vi "Fpga-FPGANic-Top.vi"() -> ()   [LabVIEW 2017]
uses:
  <instrlib>/_niInstr/Network/Ethernet/MAC/CLIP/v1/Resources.ctl
  <vilib>/Platform/TimedLoop/XDataNode/timing_clust.ctl
  <vilib>/Platform/TimedLoop/XDataNode/nitl_modes.ctl
  <vilib>/Platform/TimedLoop/XDataNode/wakeup.ctl
  FPGANic.Read.States.ctl
  <instrlib>/_niInstr/Network/Ethernet/MAC/Raw Stream/v1/niInstr Ethernet MAC Raw Stream v1.lvclass
  <instrlib>/_niInstr/Network/Ethernet/Utility/v1/FPGA/Network Data Stream.ctl
  FPGANic.Write.States.ctl
  <vilib>/rvi/Emulation/niFpgaSctlEmulationGetInTimedLoop.vi
  <vilib>/rvi/Emulation/niFpgaEmulationReportErrorSimple.vi
  <vilib>/rvi/Emulation/niFpgaGetClockAttributes.vi
  <vilib>/rvi/Emulation/niFpgaCriticalErrorInLSC.vi
  <vilib>/rvi/eio/common/nirviEmuTemplateMethod_errors.vi
  <vilib>/rvi/interface/RandomDataEmulation/niFpgaRandomDataHandleErrors.vi
  <vilib>/rvi/DataTransferAndStorage/Container/Common/niFpgaContainerGetUniqueNameForEmu.vi
  <vilib>/rvi/DataTransferAndStorage/Container/Common/niFpgaContainerSetEmuInfo.vi
  <vilib>/rvi/eio/common/nirviEmuReportErrorAndStop.vi
  <vilib>/rvi/DataTransferAndStorage/Container/Common/niFpgaContainerExecOnDevCompGetState.vi
  <vilib>/rvi/Emulation/niFpgaEmulationIsFPGAContextNoSignature.vi
  <vilib>/rvi/errors/niFpgaSetErrorForExecOnDevCompSimple.vi
  <vilib>/rvi/FIFO/Fifo_Resource/nirvififoEmulationSetSize.vi
  <vilib>/rvi/FIFO/Fifo_Resource/nirviFifoEmulationQueueMgr.vi
  <instcachedir>/0/nirviFifoEmulationQueueMgr_E5CAEC123FF24DC58D834DCA3CDAA9B5.lvgen/nirviFifoEmulationQueueMgr_E5CAEC123FF24DC58D834DCA3CDAA9B5_008.vi
  <vilib>/rvi/FIFO/Fifo_Resource/nirvififoEmulationDetermineInputValidOut.vi
  <vilib>/rvi/FIFO/Fifo_Resource/nirvififoEmulationCreateLock.vi
  <vilib>/rvi/Emulation/niFpgaProcessEmulError.vi
  <vilib>/rvi/FIFO/Fifo_Resource/nirvififoEmulationObtainLock.vi
  <vilib>/rvi/FIFO/Fifo_Resource/nirvififoEmulationReleaseLock.vi
  <vilib>/rvi/occurrence/nirviWaitOnOccurrenceBase.vi
  <vilib>/rvi/errors/nirviReportUnexpectedCaseInternalError.vi
  <vilib>/rvi/errors/nirviReportUnexpectedCaseInternalError (U32).vi
  <vilib>/Utility/error.llb/Clear Errors.vi
  <instrlib>/_niInstr/Network/Ethernet/MAC/Raw Stream/v1/Read End of Bad Frame.vi
  <instrlib>/_niInstr/Network/Ethernet/MAC/Raw Stream/v1/Read End of Good Frame.vi
  <instrlib>/_niInstr/Network/Ethernet/MAC/Raw Stream/v1/Read Data Stream.vi
  <instrlib>/_niInstr/Network/Ethernet/MAC/Raw Stream/v1/Write Data Stream.vi
  <instrlib>/_niInstr/Network/Ethernet/MAC/Raw Stream/v1/Write End of Good Frame.vi
  <vilib>/Platform/TimedLoop/XDataNode/XDataNode.xnode
  <vilib>/eio/EIONode/EIONode.xnode
  <vilib>/rvi/DataTransferAndStorage/Container/XNode/niFpgaContainer.xnode
  <vilib>/rvi/interface/RandomDataEmulation/nirviRandomDataFpgaReadWriteTemplate.vi
  <vilib>/rvi/LocalResourceManager/LocalResourceManager.xnode
  <vilib>/rvi/FIFO/Fifo_Resource/niFpgaFifoEmulationRefIn.vi
  <instrlib>/_niInstr/Network/Ethernet/MAC/CLIP/v1/niInstr Ethernet MAC - CLIP v1.lvclass
  <vilib>/Platform/TimedLoop/XDataNode/XDNodeRunTimeDep.lvlib
  <instrlib>/_niInstr/Network/Ethernet/Utility/v1/FPGA/niInstr Ethernet Utilities FPGA v1.lvlib
panel:
  in  "d_microblaze_i\\reset_rtl":bool=TRUE
  out "GPIO #1 out":u32
  in  "GPIO #1 in":u32
  in  "d_microblaze_i\\AXI_STR_RXD_3_tkeep":u8=15
  out "mgtrefclks_locked":bool
  out "mgtrefclks_valid":bool
  out "posc_complete":bool
  out "sPort0_Power_Good":bool
  out "sPort1_Power_Good":bool
  out "signal_detect_Port0":bool
  out "signal_detect_Port1":bool
  out "aBlockLockPort0":bool
  out "aBlockLockPort1":bool
  out "GPIO #2 out":u32
  in  "GPIO #2 in":u32
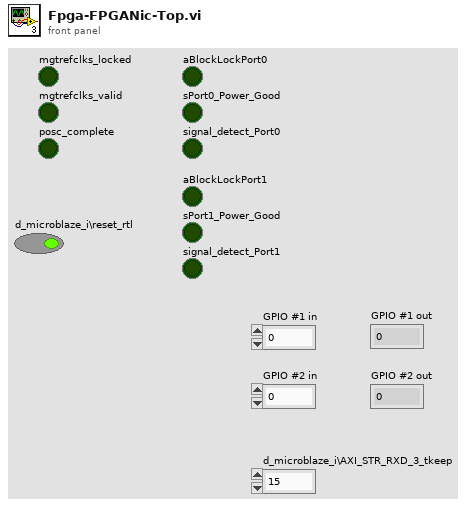
[diagram p1: front panel]
types:
  T1 = typedef "niInstr Ethernet MAC - CLIP v1.lvclass/Resources.ctl" = cluster{"RX":cluster{"TData":refnum<k21>, "TValid":refnum<k21>, "TKeep":refnum<k21>, "TLast":refnum<k21>, "TUser":refnum<k21>}, "TX":cluster{"TData":refnum<k21>, "TValid":refnum<k21>, "TKeep":refnum<k21>, "TLast":refnum<k21>, "TReady":refnum<k21>}, "Pause resources":cluster{"cPauseValuePort":refnum<k21>, "cPauseReqPort":refnum<k21>}, "MAC Clock":refnum<k21>}
  T2 = typedef "XDNodeRunTimeDep.lvlib/timing_clust.ctl" = cluster{"Expected End [f-1]":u64, "Actual End [f-1]":u64, "Finished Late? [f-1]":bool, "Expected End [i-1]":u64, "Actual End [i-1]":u64, "Finished Late? [i-1]":bool, "Expected Start [i]":u64, "Actual Start [i]":u64, "Expected Start [f]":u64, "Actual Start [f]":u64, "Source Name":string, "Structure Name":string, "Period":i64, "Deadline":i64, "Offset":i64, "Start":i64, "Priority":i32, "Timeout":i32, "Mode":T3, "Wakeup Reason":T4, "Error":errorcluster, "Source Type":string, "Secondary Source Type":string, "Global End Time":u64, "Global Start Time":u64, "Frame Duration":u64, "Iteration Duration":u64, "Assigned CPU":i32, "I/O Scan Engine Mode":u32}
  T3 = typedef "XDNodeRunTimeDep.lvlib/nitl_modes.ctl" = enum32{"No Change", "Process missed periods, maintain original phase", "Discard missed periods, maintain original phase", "Process missed periods, ignore original phase", "Discard missed periods, ignore original phase"}
  T4 = typedef "XDNodeRunTimeDep.lvlib/wakeup.ctl" = enum32{"Normal", "Aborted", "Asynchronous wakeup", "Timing source error", "Timed loop error", "Timeout"}
  T5 = typedef "niInstr Ethernet Utilities FPGA v1.lvlib/Network Data Stream.ctl" = cluster{"data":u8[], "data valid":bool, "byte enables":bool[]}
  T6 = cluster{"tdata[63:0]":u64, "tlast":bool, "tkeep[7:0]":bool[], "EndOfGoodFrame":bool, "EndOfBadFrame":bool}
  T7 = typedef "FPGANic.Write.States.ctl" = enum16{"Read-Top", "Read-Bottom"}
  T8 = typedef "FPGANic.Read.States.ctl" = enum16{"Read-Top", "Read-Bottom", "Append-Size"}
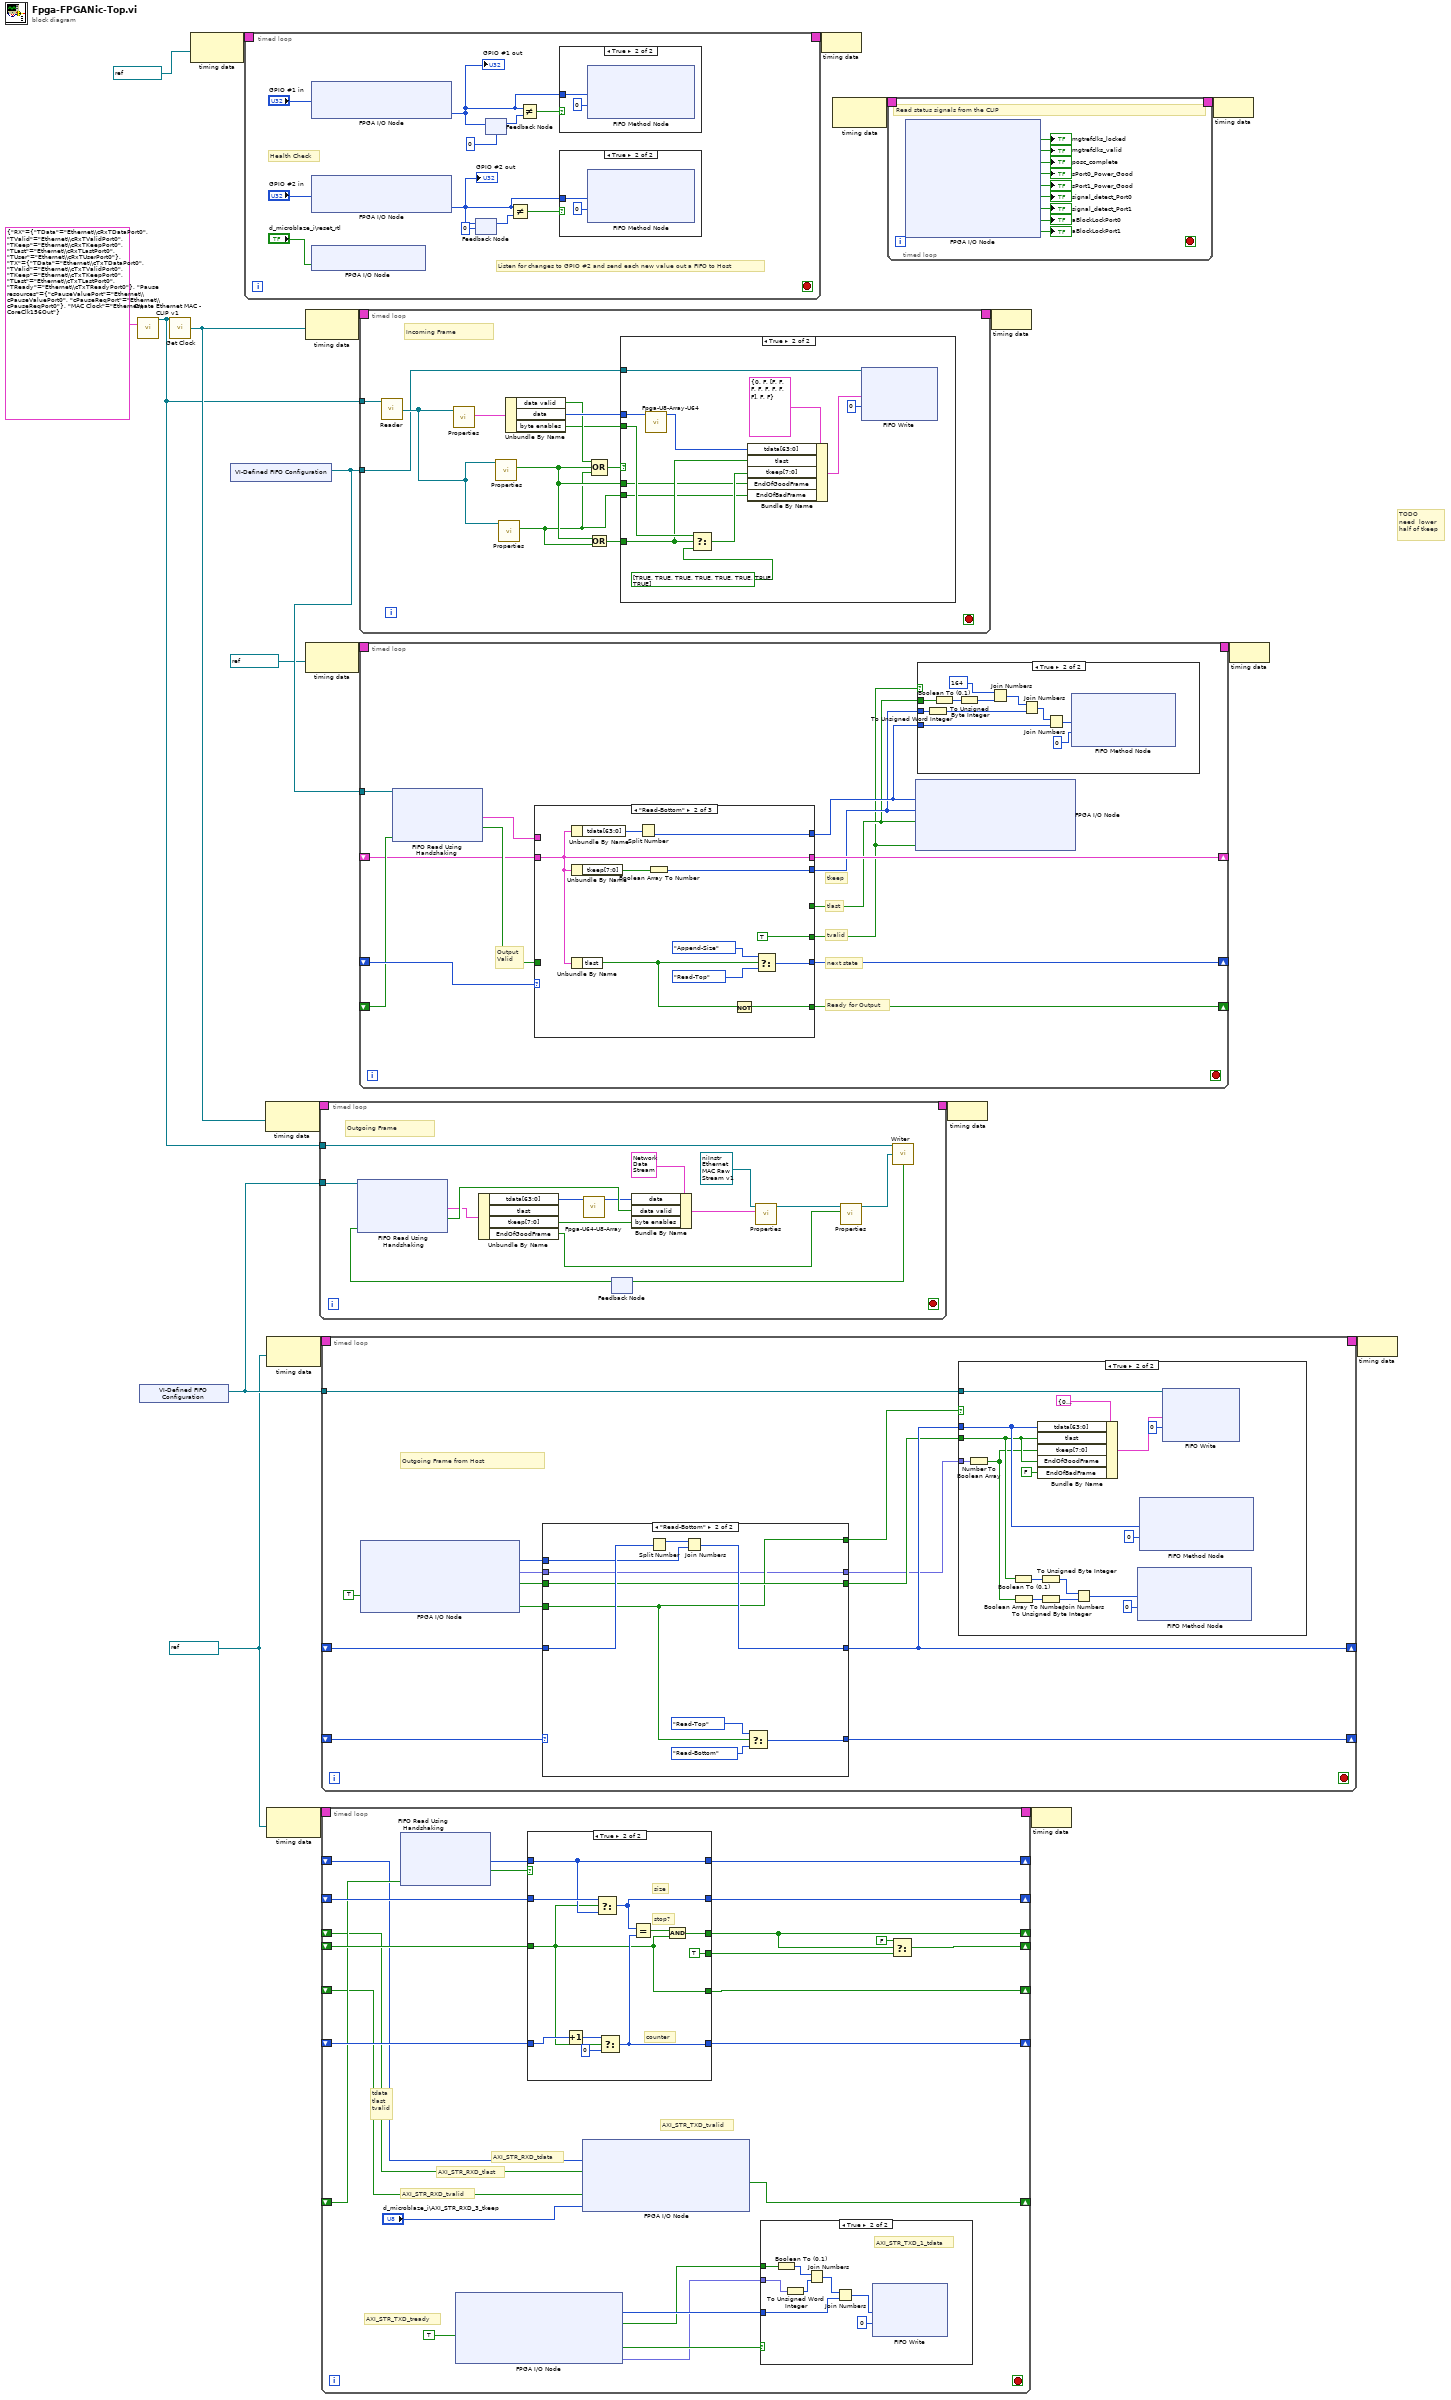
[diagram p0: block diagram]
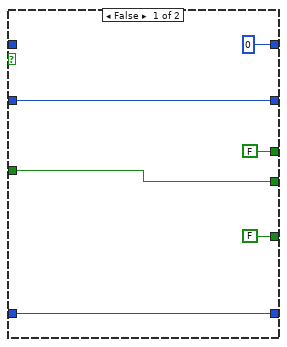
[diagram p3: hidden frame]
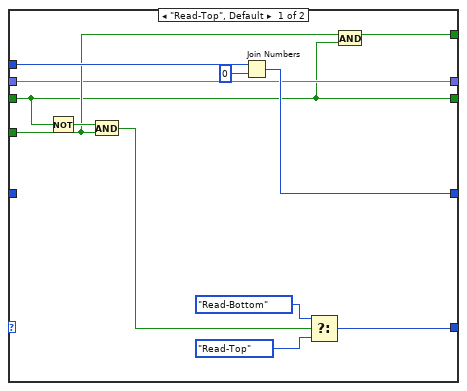
[diagram p4: hidden frame]
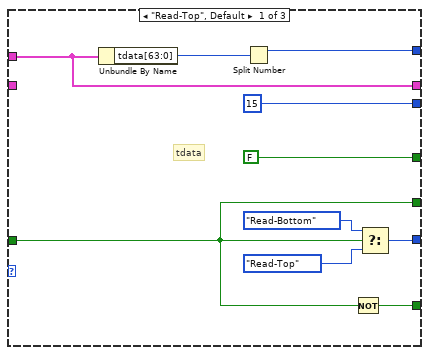
[diagram p6: hidden frame]
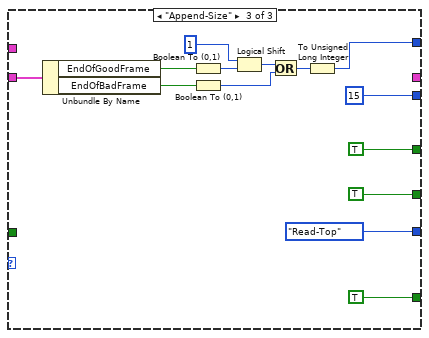
[diagram p7: hidden frame]
diagram:
  w1 = refnum<k21> "100MHz" ("Source Name")
  # "TODO\nneed  lower\nhalf of tkeep"
  n1 = call <instrlib>:"Create Ethernet MAC - CLIP v1.vi"("Ethernet AXI4-S Resources"=T1 {"RX"={"TData"="Ethernet\\cRxTDataPort0", "TValid"="Ethernet\\cRxTValidPort0", "TKeep"="Ethernet\\cRxTKeepPort0", "TLast"="Ethernet\\cRxTLastPort0", "TUser"="Ethernet\\cRxTUserPort0"}, "TX"={"TData"="Ethernet\\cTxTDataPort0", "TValid"="Ethernet\\cTxTValidPort0", "TKeep"="Ethernet\\cTxTKeepPort0", "TLast"="Ethernet\\cTxTLastPort0", "TReady"="Ethernet\\cTxTReadyPort0"}, "Pause resources"={"cPauseValuePort"="Ethernet\\cPauseValuePort0", "cPauseReqPort"="Ethernet\\cPauseReqPort0"}, "MAC Clock"="Ethernet\\CoreClk156Out"}) -> ("niInstr Ethernet MAC - CLIP v1.lvclass out"=w11:refnum<class "niInstr Ethernet MAC - CLIP v1.lvclass">)  [unwired: 14 in]
  n2 = xnode "VI-Defined FIFO Configuration"() -> ("FIFO Out"=w4:refnum<k21>)
  n3 = call-dynamic "Get Clock.vi"("niInstr Ethernet MAC - CLIP v1.lvclass"=w11) -> ("MAC Clock"=w12:refnum<k21>)  [unwired: 14 in]
  n4 = node-c288(refnum<k21> "100MHz" ("Source Name")) -> (w22:T2)
  n5 = xnode "VI-Defined FIFO Configuration"() -> ("FIFO Out"=w8:refnum<k21>)
  n6 = timed-loop {
    timing: w22 -> [_]
    timing-out: [_] -> w21
    stop <- _ stop-if-true
    # "Health Check"
    # "Listen for changes to GPIO #2 and send each new value out a FIFO to Host"
    n7 = xnode "FPGA I/O Node"("d_microblaze_i\\gpio_rtl_tri_i"="GPIO #1 in") -> ("d_microblaze_i\\gpio_rtl_0_tri_o"=w25:u32)  [unwired: 2 in, 2 out]
    "GPIO #1 out" <- w25
    n8 = xnode "FPGA I/O Node"("d_microblaze_i\\gpio_rtl_1_tri_i"="GPIO #2 in") -> ("d_microblaze_i\\gpio_rtl_2_tri_o"=w27:u32)  [unwired: 2 in, 2 out]
    "GPIO #2 out" <- w27
    n9 = xnode "FPGA I/O Node"("d_microblaze_i\\reset_rtl"="d_microblaze_i\\reset_rtl") -> ()  [unwired: 1 in, 1 out]
    n10 = feedback-in #1(w27) -> ()
    n11 = feedback #1(u32 0 ("d_microblaze_i\\gpio_rtl_2_tri_o")) -> (w32:u32)
    n12 = feedback #2(u32 0 ("d_microblaze_i\\gpio_rtl_0_tri_o")) -> (w30:u32)
    n13 = feedback-in #2(w25) -> ()
    n14 = Not Equal?(x=w27, y=w32) -> (x != y?=w29:bool)
    n15 = Not Equal?(x=w25, y=w30) -> (x != y?=w26:bool)
    n16 = case shown="True" w26 {
      tunnel: w25 -> [_ w35]
      frame False {
      }
      frame True {
        n17 = xnode ("FIFO Method Node")("Element"=w35, "Timeout"=0) -> ()  [unwired: 1 in, 2 out]
      }
    }
    n18 = case shown="True" w29 {
      tunnel: w27 -> [_ w37]
      frame False {
      }
      frame True {
        n19 = xnode ("FIFO Method Node")("Element"=w37, "Timeout"=0) -> ()  [unwired: 1 in, 2 out]
      }
    }
  }
  n20 = node-c288(w12) -> (w15:T2)
  n21 = node-c288(w1) -> (w6:T2)
  n22 = node-c288(w1) -> (w3:T2)
  n23 = node-c288(w12) -> (w19:T2)
  n24 = node-c288(refnum<k21> "100MHz" ("Source Name")) -> (w10:T2)
  n25 = timed-loop {
    timing: w15 -> [_]
    timing-out: [_] -> w14
    tunnel: w11 -> [w54]
    tunnel: w4 -> [w48]
    stop <- _ stop-if-true
    # "Outgoing Frame"
    n26 = feedback #3() -> (w47:bool)  [unwired: 1 in]
    n27 = xnode ("FIFO Read Using Handshaking")("Ready for Output"=w47, "FIFO In"=w48) -> ("Element"=w44:T6, "Output Valid"=w45:bool)  [unwired: 1 out]
    n28 = Unbundle By Name(w44) -> ("tdata[63:0]"=w41:u64, "tkeep[7:0]"=w42:bool[], "EndOfGoodFrame"=w43:bool)  [unwired: 1 out]
    n29 = call "Fpga-U64-U8-Array.vi"("U64 in"=w41) -> ("U8[] out"=w40:u8[])  [unwired: 10 in]
    n30 = Bundle By Name(cluster=T5 {"data"=[0, 0, 0, 0, 0, 0, 0, 0], "data valid"=FALSE, "byte enables"=[FALSE, FALSE, FALSE, FALSE, FALSE, FALSE, FALSE, FALSE]} ("Data Stream"), "data"=w40, "data valid"=w45, "byte enables"=w42) -> (w52:T5)
    n31 = call-poly <instrlib>:"Properties.vi"("Data Stream"=w52, "niInstr Ethernet MAC Data Stream v1 in"=refnum<class "niInstr Ethernet MAC Raw Stream v1.lvclass"> refnum) -> ("niInstr Ethernet MAC Data Stream v1 out"=w51:refnum<class "niInstr Ethernet MAC Raw Stream v1.lvclass">)  [unwired: 9 in]
    n32 = call-poly <instrlib>:"Properties.vi"("End of Good Frame"=w43, "niInstr Ethernet MAC Data Stream v1 in"=w51) -> ("niInstr Ethernet MAC Data Stream v1 out"=w49:refnum<class "niInstr Ethernet MAC Raw Stream v1.lvclass">)  [unwired: 9 in]
    n33 = call-dynamic "Writer.vi"("niInstr Ethernet MAC v1.lvclass"=w54, "niInstr Ethernet MAC Raw Stream v1.lvclass"=w49) -> ("ready for input?"=w46:bool)  [unwired: 12 in, 1 out]
    n34 = feedback-in #3(w46) -> ()
  }
  n35 = timed-loop {
    timing: w6 -> [_]
    timing-out: [_] -> w5
    tunnel: w4 -> [w68]
    shift-right: [w66] -> _
    shift-left: _ -> [w67]
    shift-right: [w61] -> _
    shift-left: _ -> [w62]
    stop <- _ stop-if-true
    # "Outgoing Frame from Host"
    n36 = xnode "FPGA I/O Node"("d_microblaze_i\\AXI_STR_TXD_tready"=TRUE ("d_microblaze_i\\AXI_STR_TXD_2_tready")) -> ("d_microblaze_i\\AXI_STR_TXD_tdata"=w65:u32, "d_microblaze_i\\AXI_STR_TXD_tkeep"=w58:fxp<+,4,4>, "d_microblaze_i\\AXI_STR_TXD_tlast"=w63:bool, "d_microblaze_i\\AXI_STR_TXD_tvalid"=w64:bool)  [unwired: 5 in, 5 out]
    n37 = case shown="\"Read-Bottom\"" w67 {
      tunnel: [w79 w89] -> w66
      tunnel: w65 -> [w78 w85]
      tunnel: w64 -> [w73 w83]
      tunnel: [w76 w88] -> w61
      tunnel: w63 -> [w70 w84]
      tunnel: [w70 w84] -> w60
      tunnel: w62 -> [_ w87]
      tunnel: [w71 w83] -> w59
      tunnel: w58 -> [w72 w82]
      tunnel: [w72 w82] -> w57
      frame "Read-Top", Default {
        n38 = Not(x=w70) -> (.not. x?=w75:bool)
        n39 = And(x=w75, y=w73) -> (x .and. y?=w74:bool)
        n40 = Join Numbers(hi=w78, lo=u32 0) -> ((hi.lo)=w76:u64)
        n41 = Select(t=FPGANic.Write.States."Read-Bottom" ("Enum"), s=w74, f=FPGANic.Write.States."Read-Top" ("Enum")) -> (s? t:f=w79:T7)
        n42 = And(x=w73, y=w70) -> (x .and. y?=w71:bool)
      }
      frame "Read-Bottom" {
        n43 = Split Number(x=w87) -> (hi(x)=w86:u32)  [unwired: 1 out]
        n44 = Join Numbers(hi=w86, lo=w85) -> ((hi.lo)=w88:u64)
        n45 = Select(t=FPGANic.Write.States."Read-Top" ("Enum"), s=w83, f=FPGANic.Write.States."Read-Bottom" ("Enum")) -> (s? t:f=w89:T7)
      }
    }
    n46 = case shown="True" w59 {
      tunnel: w68 -> [_ w107]
      tunnel: w61 -> [_ w102]
      tunnel: w60 -> [_ w99]
      tunnel: w57 -> [_ w106]
      frame False {
      }
      frame True {
        n47 = Number To Boolean Array(number=w106) -> (Boolean array=w95:bool[])
        n48 = Boolean To (0,1)(Boolean=w99) -> (0, 1=w97:i16)
        n49 = Boolean Array To Number(Boolean array=w95) -> (number=w94:u8)
        n50 = Bundle By Name(cluster=T6 {"tdata[63:0]"=0, "tlast"=FALSE, "tkeep[7:0]"=[FALSE, FALSE, FALSE, FALSE, FALSE, FALSE, FALSE, FALSE], "EndOfGoodFrame"=FALSE, "EndOfBadFrame"=FALSE} ("AXI4-Pins"), "tdata[63:0]"=w102, "tlast"=w99, "tkeep[7:0]"=w95, "EndOfGoodFrame"=w99, "EndOfBadFrame"=FALSE) -> (w104:T6)
        n51 = To Unsigned Byte Integer(number=w97) -> (unsigned 8bit integer=w96:u8)
        n52 = To Unsigned Byte Integer(number=w94) -> (unsigned 8bit integer=w93:u8)
        n53 = Join Numbers(hi=w96, lo=w93) -> ((hi.lo)=w98:u16)
        n54 = xnode ("FIFO Method Node")("Element"=w98, "Timeout"=0) -> ()  [unwired: 1 in, 2 out]
        n55 = xnode ("FIFO Method Node")("Element"=w102, "Timeout"=0) -> ()  [unwired: 1 in, 2 out]
        n56 = xnode ("FIFO Write")("Element"=w104, "Timeout"=0, "FIFO In"=w107) -> ()  [unwired: 2 out]
      }
    }
  }
  n57 = timed-loop {
    timing: w3 -> [_]
    timing-out: [_] -> w2
    shift-right: [w116] -> _
    shift-left: _ -> [w132]
    shift-right: [w129] -> _
    shift-left: _ -> [w131]
    shift-right: [w127] -> _
    shift-left: _ -> [w128]
    shift-right: [w114] -> _
    shift-left: _ -> [w122]
    shift-right: [w113] -> _
    shift-left: _ -> [w126]
    shift-right: [w125] -> _
    shift-left: _ -> [w124]
    shift-right: [w115] -> _
    shift-left: _ -> [w123]
    stop <- _ stop-if-true
    # "AXI_STR_TXD_tvalid"
    # "AXI_STR_TXD_tready"
    # "AXI_STR_RXD_tvalid"
    # "AXI_STR_RXD_tlast"
    # "AXI_STR_RXD_tdata"
    # "tdata\ntlast\ntvalid"
    n58 = xnode ("FIFO Read Using Handshaking")("Ready for Output"=w126) -> ("Element"=w130:u64, "Output Valid"=w133:bool)  [unwired: 1 in, 1 out]
    n59 = xnode "FPGA I/O Node"("d_microblaze_i\\AXI_STR_TXD_1_tready"=TRUE ("d_microblaze\\AXI_STR_TXD_tready")) -> ("d_microblaze_i\\AXI_STR_TXD_1_tdata"=w119:u32, "d_microblaze_i\\AXI_STR_TXD_1_tlast"=w111:bool, "d_microblaze_i\\AXI_STR_TXD_1_tvalid"=w120:bool, "d_microblaze_i\\AXI_STR_TXD_1_tkeep"=w110:fxp<+,4,4>)  [unwired: 5 in, 5 out]
    n60 = case shown="True" w133 {
      tunnel: w132 -> [w146 w148]
      tunnel: [w146 TRUE ("Size\nRead?")] -> w117
      tunnel: w131 -> [w147 w158]
      tunnel: w130 -> [_ w153]
      tunnel: [w147 w152] -> w129
      tunnel: w128 -> [w145 w157]
      tunnel: [w145 w151] -> w127
      tunnel: [FALSE ("Size\nRead?") w148] -> w114
      tunnel: [u32 0 ("Element") w153] -> w125
      tunnel: [FALSE w149] -> w115
      frame False {
      }
      frame True {
        # "stop?"
        # "size"
        # "counter"
        n61 = Increment(x=w157) -> (x+1=w155:u32)
        n62 = Select(t=w158, s=w148, f=w153) -> (s? t:f=w152:u64)
        n63 = Select(t=w155, s=w148, f=u32 0) -> (s? t:f=w151:u32)
        n64 = Equal?(x=w152, y=w151) -> (x = y?=w150:bool)
        n65 = And(x=w150, y=w148) -> (x .and. y?=w149:bool)
      }
    }
    n66 = xnode "FPGA I/O Node"("d_microblaze_i\\AXI_STR_RXD_1_tdata"=w124, "d_microblaze_i\\AXI_STR_RXD_1_tlast"=w123, "d_microblaze_i\\AXI_STR_RXD_1_tvalid"=w122, "d_microblaze_i\\AXI_STR_RXD_1_tkeep"="d_microblaze_i\\AXI_STR_RXD_3_tkeep") -> ("d_microblaze_i\\AXI_STR_RXD_1_tready"=w113:bool)  [unwired: 5 in, 5 out]
    n67 = case shown="True" w120 {
      tunnel: w119 -> [_ w140]
      tunnel: w111 -> [_ w136]
      tunnel: w110 -> [_ w135]
      frame False {
      }
      frame True {
        # "AXI_STR_TXD_1_tdata"
        n68 = Boolean To (0,1)(Boolean=w136) -> (0, 1=w137:i16)
        n69 = To Unsigned Word Integer(number=w135) -> (unsigned 16bit integer=w134:u16)
        n70 = Join Numbers(hi=w137, lo=w134) -> ((hi.lo)=w138:u32)
        n71 = Join Numbers(hi=w138, lo=w140) -> ((hi.lo)=w139:u64)
        n72 = xnode ("FIFO Write")("Element"=w139, "Timeout"=0) -> ()  [unwired: 1 in, 2 out]
      }
    }
    n73 = Select(t=FALSE, s=w115, f=w117) -> (s? t:f=w116:bool)
  }
  n74 = timed-loop {
    timing: w19 -> [_]
    timing-out: [_] -> w18
    tunnel: w11 -> [w171]
    tunnel: w8 -> [w167]
    stop <- _ stop-if-true
    # "Incoming Frame"
    n75 = call-dynamic "Reader.vi"("niInstr Ethernet MAC - CLIP v1.lvclass 2"=w171) -> ("niInstr Ethernet MAC Raw Stream v1.lvclass"=w168:refnum<class "niInstr Ethernet MAC Raw Stream v1.lvclass">)  [unwired: 13 in, 1 out]
    n76 = call-poly <instrlib>:"Properties.vi"("niInstr Ethernet MAC Data Stream v1 in"=w168) -> ("Data Stream"=w170:T5)  [unwired: 9 in, 1 out]
    n77 = call-poly <instrlib>:"Properties.vi"("niInstr Ethernet MAC Data Stream v1 in"=w168) -> ("End of Good Frame"=w162:bool)  [unwired: 9 in, 1 out]
    n78 = call-poly <instrlib>:"Properties.vi"("niInstr Ethernet MAC Data Stream v1 in"=w168) -> ("End of Bad Frame"=w161:bool)  [unwired: 9 in, 1 out]
    n79 = Unbundle By Name(w170) -> ("data valid"=w166:bool, "data"=w169:u8[], "byte enables"=w163:bool[])
    n80 = Or(x=w162, y=w161) -> (x .or. y?=w164:bool)
    n81 = Compound Arithmetic op=OR(w166, w162, w161) -> (w165:bool)
    n82 = case shown="True" w165 {
      tunnel: w169 -> [_ w181]
      tunnel: w167 -> [_ w182]
      tunnel: w164 -> [_ w175]
      tunnel: w163 -> [_ w176]
      tunnel: w162 -> [_ w174]
      tunnel: w161 -> [_ w173]
      frame False {
      }
      frame True {
        n83 = call "Fpga-U8-Array-U64.vi"("U8[] in"=w181) -> ("U64 out"=w178:u64)  [unwired: 10 in]
        n84 = Select(t=w176, s=w175, f=bool[] [TRUE, TRUE, TRUE, TRUE, TRUE, TRUE, TRUE, TRUE] ("s? t:f")) -> (s? t:f=w177:bool[])
        n85 = Bundle By Name(cluster=T6 {"tdata[63:0]"=0, "tlast"=FALSE, "tkeep[7:0]"=[FALSE, FALSE, FALSE, FALSE, FALSE, FALSE, FALSE, FALSE], "EndOfGoodFrame"=FALSE, "EndOfBadFrame"=FALSE} ("Element"), "tdata[63:0]"=w178, "tlast"=w175, "tkeep[7:0]"=w177, "EndOfGoodFrame"=w174, "EndOfBadFrame"=w173) -> (w179:T6)
        n86 = xnode ("FIFO Write")("Element"=w179, "Timeout"=0, "FIFO In"=w182) -> ()  [unwired: 2 out]
      }
    }
  }
  n87 = timed-loop {
    timing: w10 -> [_]
    timing-out: [_] -> w9
    tunnel: w8 -> [w198]
    shift-right: [w195] -> _
    shift-left: _ -> [w190]
    shift-right: [w194] -> _
    shift-left: _ -> [w193]
    shift-right: [w192] -> _
    shift-left: _ -> [w191]
    stop <- _ stop-if-true
    # "Output\nValid"
    # "Ready for Output"
    # "next state"
    # "tkeep"
    # "tlast"
    # "tvalid"
    n88 = xnode ("FIFO Read Using Handshaking")("Ready for Output"=w191, "FIFO In"=w198) -> ("Element"=w196:T6, "Output Valid"=w197:bool)  [unwired: 1 out]
    n89 = case shown="\"Read-Bottom\"" w193 {
      tunnel: w197 -> [w200 _ _]
      tunnel: w196 -> [w201 _ _]
      tunnel: [w207 w218 w224] -> w189
      tunnel: [w204 w214 FPGANic.Read.States."Read-Top" ("Enum")] -> w194
      tunnel: [w200 TRUE ("Output Valid") TRUE ("Output Valid")] -> w186
      tunnel: [FALSE _ TRUE] -> w187
      tunnel: [u8 15 ("t") w216 u8 15 ("t")] -> w188
      tunnel: [w201 w215 _] -> w195
      tunnel: [w199 w209 TRUE ("tlast")] -> w192
      tunnel: w190 -> [_ w215 w227]
      frame "Read-Top", Default {
        # "tdata"
        n90 = Unbundle By Name(w201) -> ("tdata[63:0]"=w208:u64)
        n91 = Split Number(x=w208) -> (hi(x)=w207:u32)  [unwired: 1 out]
        n92 = Not(x=w200) -> (.not. x?=w199:bool)
        n93 = Select(t=FPGANic.Read.States."Read-Bottom" ("Enum"), s=w200, f=FPGANic.Read.States."Read-Top" ("Enum")) -> (s? t:f=w204:T8)
      }
      frame "Read-Bottom" {
        n94 = Unbundle By Name(w215) -> ("tdata[63:0]"=w219:u64)
        n95 = Unbundle By Name(w215) -> ("tkeep[7:0]"=w217:bool[])
        n96 = Unbundle By Name(w215) -> ("tlast"=w211:bool)
        n97 = Split Number(x=w219) -> (lo(x)=w218:u32)  [unwired: 1 out]
        n98 = Boolean Array To Number(Boolean array=w217) -> (number=w216:u8)
        n99 = Not(x=w211) -> (.not. x?=w209:bool)
        n100 = Select(t=FPGANic.Read.States."Append-Size" ("Enum"), s=w211, f=FPGANic.Read.States."Read-Top" ("Enum")) -> (s? t:f=w214:T8)
      }
      frame "Append-Size" {
        n101 = Unbundle By Name(w227) -> ("EndOfGoodFrame"=w226:bool, "EndOfBadFrame"=w225:bool)
        n102 = Boolean To (0,1)(Boolean=w226) -> (0, 1=w231:i16)
        n103 = Boolean To (0,1)(Boolean=w225) -> (0, 1=w228:i16)
        n104 = Logical Shift(y=i16 1, x=w231) -> (x << y=w229:i16)
        n105 = Or(x=w229, y=w228) -> (x .or. y?=w232:i16)
        n106 = To Unsigned Long Integer(number=w232) -> (unsigned 32bit integer=w224:u32)
      }
    }
    n107 = xnode "FPGA I/O Node"("d_microblaze_i\\AXI_STR_RXD_tdata"=w189, "d_microblaze_i\\AXI_STR_RXD_tkeep"=w188, "d_microblaze_i\\AXI_STR_RXD_tlast"=w187, "d_microblaze_i\\AXI_STR_RXD_tvalid"=w186) -> ()  [unwired: 5 in, 6 out]
    n108 = case shown="True" w186 {
      tunnel: w189 -> [_ w242]
      tunnel: w188 -> [_ w241]
      tunnel: w187 -> [_ w239]
      frame False {
      }
      frame True {
        n109 = To Unsigned Word Integer(number=w241) -> (unsigned 16bit integer=w237:u16)
        n110 = Boolean To (0,1)(Boolean=w239) -> (0, 1=w238:i16)
        n111 = To Unsigned Byte Integer(number=w238) -> (unsigned 8bit integer=w236:u8)
        n112 = Join Numbers(hi=u8 164, lo=w236) -> ((hi.lo)=w235:u16)
        n113 = Join Numbers(hi=w235, lo=w237) -> ((hi.lo)=w240:u32)
        n114 = Join Numbers(hi=w240, lo=w242) -> ((hi.lo)=w243:u64)
        n115 = xnode ("FIFO Method Node")("Element"=w243, "Timeout"=0) -> ()  [unwired: 1 in, 2 out]
      }
    }
  }
  n116 = node-c288(w21) -> ()
  n117 = node-c288() -> (w17:T2)  [unwired: 1 in]
  n118 = timed-loop {
    timing: w17 -> [_]
    timing-out: [_] -> w16
    stop <- _ stop-if-true
    # "Read status signals from the CLIP"
    n119 = xnode "FPGA I/O Node"() -> ("Ethernet\\MgtRefClks_Locked"=→"mgtrefclks_locked":bool, "Ethernet\\MgtRefClks_Valid"=→"mgtrefclks_valid":bool, "Ethernet\\POSC_Complete"=→"posc_complete":bool, "Ethernet\\sPort0_Power_Good"=→"sPort0_Power_Good":bool, "Ethernet\\sPort1_Power_Good"=→"sPort1_Power_Good":bool, "Ethernet\\signal_detect_Port0"=→"signal_detect_Port0":bool, "Ethernet\\signal_detect_Port1"=→"signal_detect_Port1":bool, "Ethernet\\aBlockLockPort0"=→"aBlockLockPort0":bool, "Ethernet\\aBlockLockPort1"=→"aBlockLockPort1":bool)  [unwired: 9 in, 9 out]
  }
  n120 = node-c288(w14) -> ()
  n121 = node-c288(w18) -> ()
  n122 = node-c288(w2) -> ()
  n123 = node-c288(w16) -> ()
  n124 = node-c288(w9) -> ()
  n125 = node-c288(w5) -> ()
